vi "_TEST_ObjCacher1.vi"(8 "error in (no error)":errorcluster, 11 "String":string) -> (0 "error out":errorcluster)   [LabVIEW 2017]
uses:
  439b7e7e-2de8-4b6a-ab75-8c530a1820e0.vi
  05bc4a04-b8e2-45f4-96d1-af1a84d1c08b.vi
  4984ed95-b616-47af-8191-0c57989a5f6f.vi
  d206f00a-0650-4c1f-a327-a45bdc6aed31.vi
  75cba76a-a9c1-4693-b9a2-998b49f0b81c.vi
  ae1eb475-346e-49ac-b7b2-b013fc25bb92.vi
  b8c799e4-df35-4b14-816d-139ca8e9513e.vi
  439b7e7e-2de8-4b6a-ab75-8c530a1820e0.vi/df97a732-2aa1-48ca-a021-ea6fe392e42b.vi
  05bc4a04-b8e2-45f4-96d1-af1a84d1c08b.vi/ccdad7bb-004e-4762-afb1-65ca7d6130ea.vi
  <userlib>/NEVSTOP-Programming-Palette/Application/Valid VI Reference_nevstop.vi
  4984ed95-b616-47af-8191-0c57989a5f6f.vi/b7be58e1-3d0a-4835-8841-f13dfc0f9efe.vi
  4984ed95-b616-47af-8191-0c57989a5f6f.vi/69f77548-5889-44c6-8640-e9f058736a5d.vi
  4984ed95-b616-47af-8191-0c57989a5f6f.vi/ea8d3cea-2f8d-4420-9a60-a5294947b6ae.vi
  d206f00a-0650-4c1f-a327-a45bdc6aed31.vi/ccdad7bb-004e-4762-afb1-65ca7d6130ea.vi
  75cba76a-a9c1-4693-b9a2-998b49f0b81c.vi/aaef58af-3a80-4898-9b69-f04cd84d0e55.vi
  ae1eb475-346e-49ac-b7b2-b013fc25bb92.vi/e699d232-c896-4670-a9c5-e7dd2195749c.vi
  b8c799e4-df35-4b14-816d-139ca8e9513e.vi/aaef58af-3a80-4898-9b69-f04cd84d0e55.vi
  4984ed95-b616-47af-8191-0c57989a5f6f.vi/b7be58e1-3d0a-4835-8841-f13dfc0f9efe.vi/ccdad7bb-004e-4762-afb1-65ca7d6130ea.vi
  <userlib>/_OpenG.lib/md5/md5.llb/MD5 Message Digest (Hexadecimal String)__ogtk.vi
  Data/_support/Get DataType Description String.vi
  _support/Resource.vi
  ObjectCacherAPI.lvlib
panel:
  out "element 4":string
  out "cacher 3":variant
  out "cacher":variant
  out "names":string[](array[string])
  out "element 3":string
  out "data string 3":string
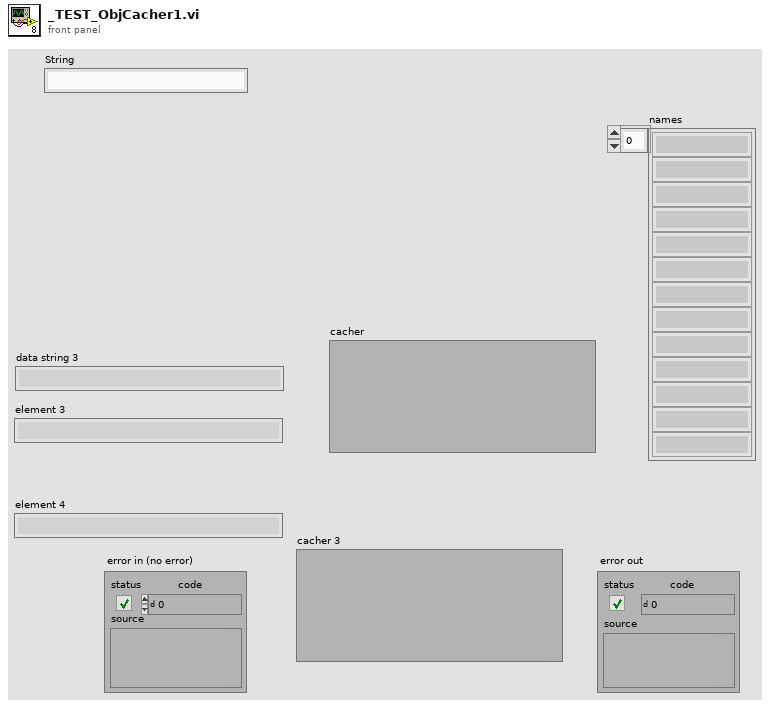
[diagram p1: front panel]
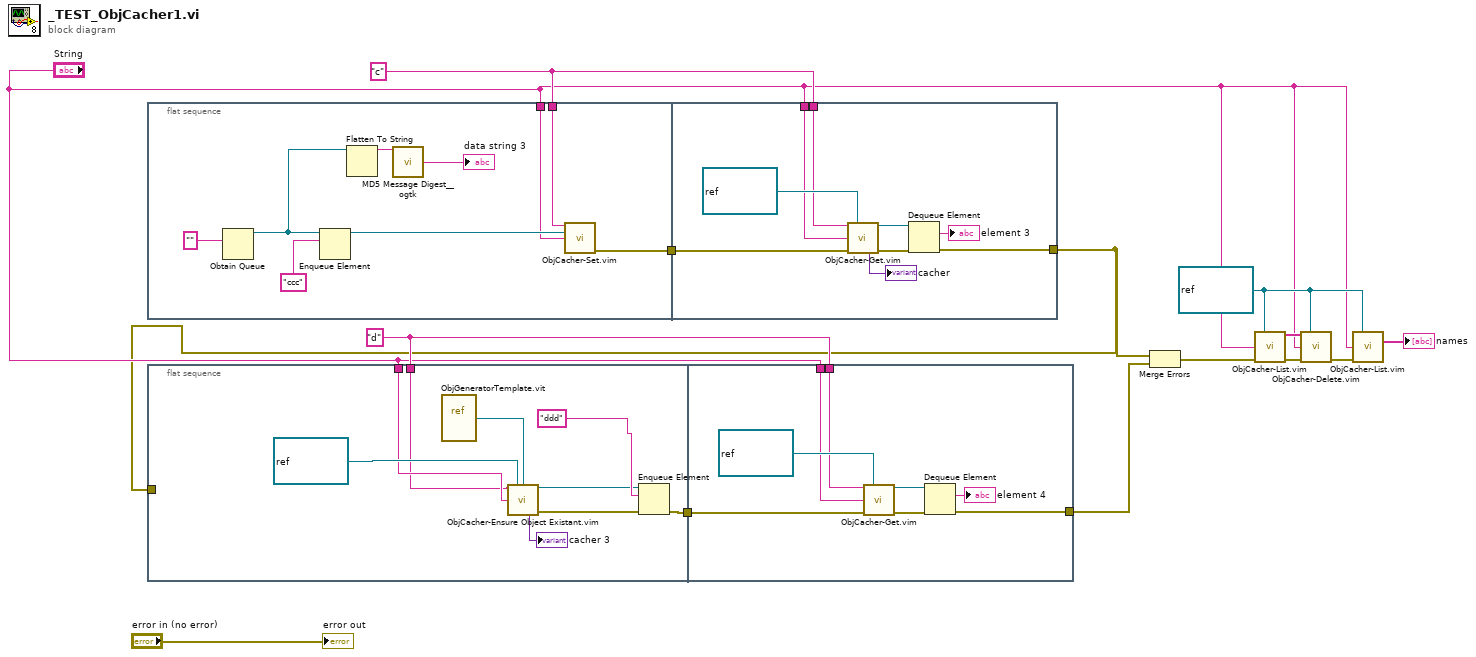
[diagram p0: block diagram]
diagram:
  w3 = "d" ("key")
  w7 = refnum<queue> refnum ("queue out")
  w13 = "c" ("key")
  n1 = flat-sequence {
    tunnel: w13 -> [w17]
    tunnel: "String" -> [w15]
    tunnel: [w16] -> w6
    tunnel: w13 -> [w29]
    tunnel: [w28] -> w1
    tunnel: "String" -> [w27]
    tunnel: w6 -> [w26]
    frame #0 {
      n2 = Obtain Queue(element data type="") -> (queue out=w21:refnum<queue>)  [unwired: 4 in, 2 out]
      n3 = Enqueue Element(queue=w21, element="ccc") -> (queue out=w18:refnum<queue>)  [unwired: 2 in, 2 out]
      n4 = Flatten To String(anything=w21) -> (data string=w20:string)  [unwired: 3 in, 2 out]
      n5 = call-poly <userlib>:"MD5 Message Digest__ogtk.vi"("Message"=w20) -> ("MD5 Message Digest"=→"data string 3":string)
      n6 = call "ObjCacher-Set.vim"("Module Name"=w17, "data"=w18, "typeKey(\"\" to use DataTypeDescription)"=w15) -> ("error out"=w16:errorcluster)  [unwired: 10 in, 2 out]
    }
    frame #1 {
      n7 = call "ObjCacher-Get.vim"("Module Name"=w29, "type"=refnum<queue> refnum ("queue out"), "typeKey(\"\" to use DataTypeDescription)"=w27, "error in (no error)"=w26) -> ("Variant"=w30:refnum<queue>, "cacher"=→"cacher":variant, "error out"=w25:errorcluster)  [unwired: 8 in, 1 out]
      n8 = Dequeue Element(queue=w30, error in (no error)=w25) -> (element=→"element 3":string, error out=w28:errorcluster)  [unwired: 1 in, 2 out]
    }
  }
  n9 = flat-sequence {
    tunnel: w3 -> [w34]
    tunnel: "String" -> [w35]
    tunnel: [w38] -> w5
    tunnel: w1 -> [_]
    tunnel: w3 -> [w46]
    tunnel: [w45] -> w4
    tunnel: "String" -> [w44]
    tunnel: w5 -> [w43]
    frame #0 {
      n10 = vi-ref "ObjGeneratorTemplate.vit"() -> (w41:refnum<vi>)
      n11 = call "ObjCacher-Ensure Object Existant.vim"("Module Name"=w34, "type"=refnum<queue> refnum ("queue out"), "Generator VI Ref"=w41, "typeKey(\"\" to use DataTypeDescription)"=w35) -> ("Variant"=w33:refnum<queue>, "cacher"=→"cacher 3":variant, "error out"=w39:errorcluster)  [unwired: 8 in, 1 out]
      n12 = Enqueue Element(queue=w33, element="ddd", error in (no error)=w39) -> (error out=w38:errorcluster)  [unwired: 1 in, 2 out]
    }
    frame #1 {
      n13 = call "ObjCacher-Get.vim"("Module Name"=w46, "type"=refnum<queue> refnum ("queue out"), "typeKey(\"\" to use DataTypeDescription)"=w44, "error in (no error)"=w43) -> ("Variant"=w47:refnum<queue>, "error out"=w42:errorcluster)  [unwired: 8 in, 2 out]
      n14 = Dequeue Element(queue=w47, error in (no error)=w42) -> (element=→"element 4":string, error out=w45:errorcluster)  [unwired: 1 in, 2 out]
    }
  }
  n15 = Merge Errors(w1, w4) -> (w12:errorcluster)
  n16 = call "ObjCacher-List.vim"("Variant"=w7, "typeKey(\"\" to use DataTypeDescription)"="String", "error in (no error)"=w12) -> ("names"=w10:string[], "error out"=w11:errorcluster)  [unwired: 9 in, 2 out]
  n17 = call "ObjCacher-Delete.vim"("Module Name"=w10, "type"=w7, "typeKey(\"\" to use DataTypeDescription)"="String", "error in (no error)"=w11) -> ("error out"=w9:errorcluster)  [unwired: 9 in, 2 out]
  n18 = call "ObjCacher-List.vim"("Variant"=w7, "typeKey(\"\" to use DataTypeDescription)"="String", "error in (no error)"=w9) -> ("names"=→"names":string[])  [unwired: 9 in, 3 out]
  "error out" <- "error in (no error)"
